vi "Sweep_Process.vi"(8 "错误输入（无错误）":errorcluster, 9 "MPM":refnum<k24>[](array[refnum]), 10 "TSL":refnum<k24>, 11 "SPU":refnum<k24>) -> (0 "error out":errorcluster, 1 "MPM out":refnum<k24>[](array[refnum]), 2 "TSL out":refnum<k24>, 3 "SPU out":refnum<k24>)   [LabVIEW 2017]
doc: "Sweep"
uses:
  D:/test/ILSTS/LV_IL/LV_IL_Sample_x64/DLL/InstrumentDLL.dll
  DLL/InstrumentDLL.dll
  Share/PowerMonitorType.vi
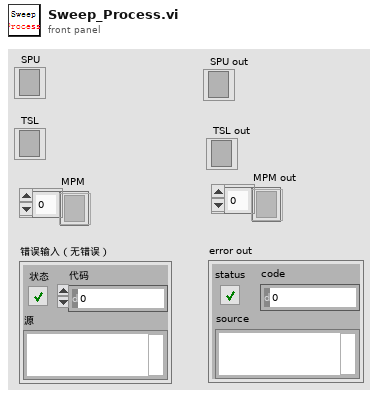
[diagram p1: front panel]
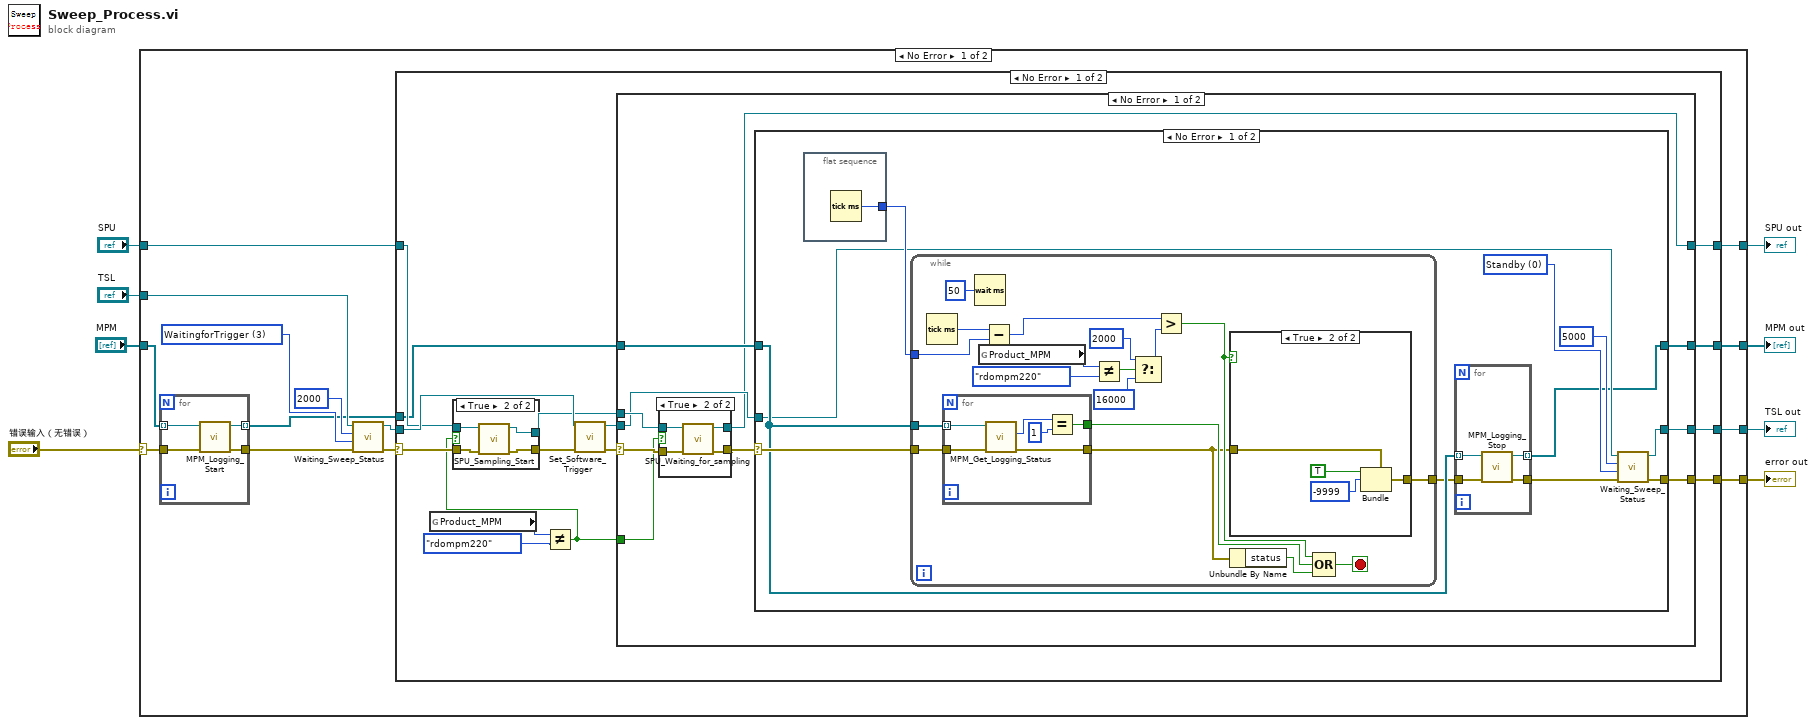
[diagram p0: block diagram]
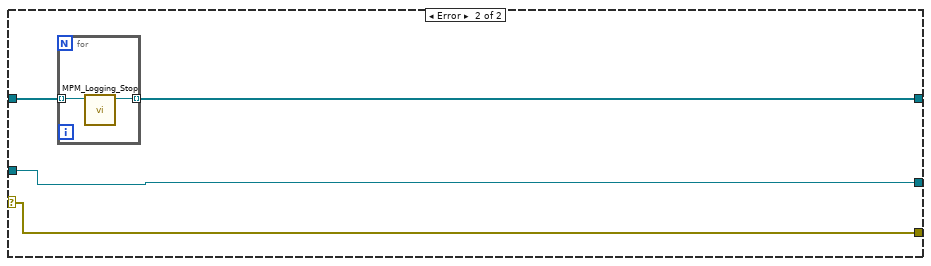
[diagram p5: hidden frame]
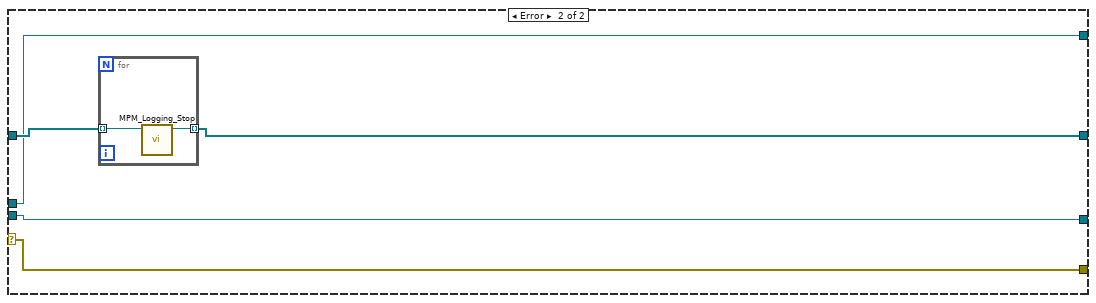
[diagram p6: hidden frame]
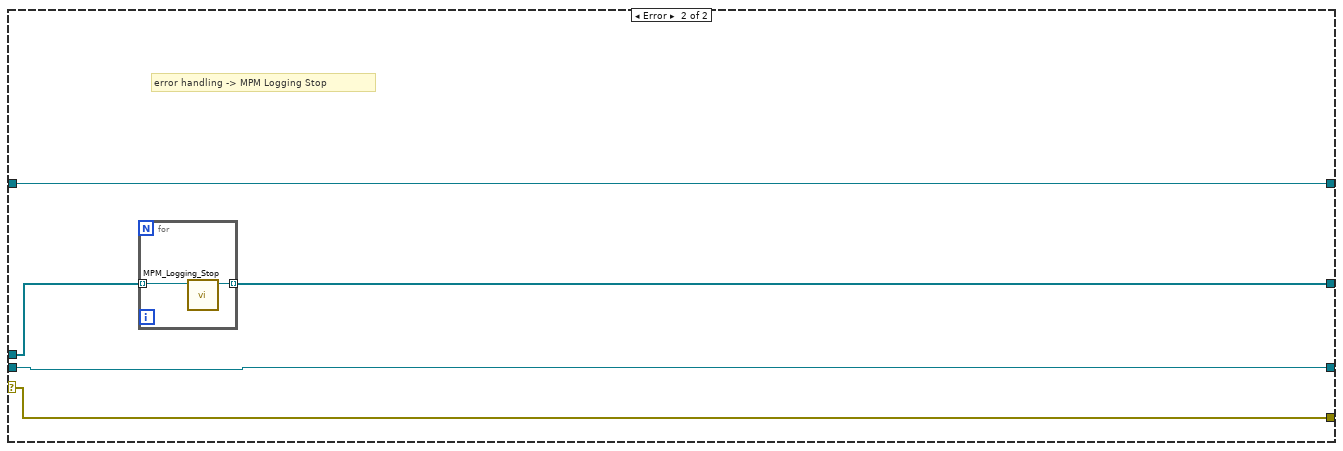
[diagram p7: hidden frame]
diagram:
  n1 = case shown="No Error" "错误输入（无错误）" {
    selector: "错误输入（无错误）" -> [w13 w132]
    tunnel: "SPU" -> [w22 w131]
    tunnel: "TSL" -> [w16 w130]
    tunnel: [w15 w132] -> w6
    tunnel: "MPM" -> [w14 w129]
    tunnel: [w12 w131] -> w3
    tunnel: [w11 w130] -> w2
    tunnel: [w9 w129] -> w1
    frame No Error {
      w19 = 3 items=["Standby", "Running", "Pausing", "WaitingforTrigger", "Returning"] ("status")
      n2 = for {
        tunnel: w14 -> [w128] mode=indexing
        tunnel: w13 -> [w127]
        tunnel: [w126] -> w17
        tunnel: [w125] -> w10 mode=indexing
        n3 = call "MPM_Logging_Start.vi"("error in (no error)"=w127, ".NET Reference in"=w128) -> ("error out"=w126:errorcluster, "Reference out"=w125:refnum<k24>)  [unwired: 8 in]
      }
      n4 = call "Waiting_Sweep_Status.vi"("error in (no error)"=w17, "status"=w19, "Wait time(msec)"=2000, ".NET Reference in"=w16) -> ("error out"=w20:errorcluster, "Reference out"=w21:refnum<k24>)  [unwired: 6 in]
      n5 = case shown="No Error" w20 {
        selector: w20 -> [w35 w121]
        tunnel: w21 -> [w36 w118]
        tunnel: w22 -> [w34 w120]
        tunnel: w10 -> [w33 w122]
        tunnel: [w29 w121] -> w15
        tunnel: [w28 w120] -> w12
        tunnel: [w27 w118] -> w11
        tunnel: [w26 w119] -> w9
        frame No Error {
          n6 = global read "PowerMonitorType.vi" "Product_MPM"() -> (w25:enum32{"rdompm210", "rdompm220"})
          n7 = Not Equal?(x=w25, y=enum32{"rdompm210", "rdompm220"}."rdompm220") -> (x != y?=w23:bool)
          n8 = case shown="True" w23 {
            tunnel: [w38 w43] -> w37
            tunnel: w35 -> [w38 w42]
            tunnel: w34 -> [w39 w41]
            tunnel: [w39 w40] -> w31
            frame False {
            }
            frame True {
              n9 = call "SPU_Sampling_Start.vi"("错误输入（无错误）"=w42, "引用"=w41) -> ("error IO"=w43:errorcluster, "引用输出"=w40:refnum<k24>)  [unwired: 7 in]
            }
          }
          n10 = call "Set_Software_Trigger.vi"("error in (no error)"=w37, ".NET Reference in"=w36) -> ("error out"=w32:errorcluster, "Reference out"=w30:refnum<k24>)  [unwired: 8 in]
          n11 = case shown="No Error" w32 {
            selector: w32 -> [w53 w114]
            tunnel: w33 -> [w50 w115]
            tunnel: w31 -> [w52 w113]
            tunnel: w30 -> [w49 w111]
            tunnel: [w48 w114] -> w29
            tunnel: [w47 w113] -> w28
            tunnel: [w46 w111] -> w27
            tunnel: [w45 w112] -> w26
            tunnel: w23 -> [w44 _]
            frame No Error {
              n12 = case shown="True" w44 {
                tunnel: w53 -> [w54 w59]
                tunnel: w52 -> [w55 w58]
                tunnel: [w54 w57] -> w51
                tunnel: [w55 w56] -> w47
                frame False {
                }
                frame True {
                  n13 = call "SPU_Waiting_for_sampling.vi"("错误输入（无错误）"=w59, "引用"=w58) -> ("error IO"=w57:errorcluster, "引用输出"=w56:refnum<k24>)  [unwired: 7 in]
                }
              }
              n14 = case shown="No Error" w51 {
                selector: w51 -> [w70 w107]
                tunnel: w50 -> [w68 w108]
                tunnel: w49 -> [w64 w105]
                tunnel: [w63 w107] -> w48
                tunnel: [w61 w105] -> w46
                tunnel: [w60 w106] -> w45
                frame No Error {
                  w66 = 0 items=["Standby", "Running", "Pausing", "WaitingforTrigger", "Returning"] ("status")
                  n15 = flat-sequence {
                    tunnel: [w75] -> w69
                    frame #0 {
                      n16 = Tick Count (ms)() -> (millisecond timer value=w75:u32)
                    }
                  }
                  n17 = while {
                    tunnel: w68 -> [w93]
                    tunnel: w70 -> [w92]
                    tunnel: w69 -> [w89]
                    tunnel: [w82] -> w62
                    stop <- w86 stop-if-true
                    n18 = Tick Count (ms)() -> (millisecond timer value=w90:u32)
                    n19 = for {
                      tunnel: w93 -> [w104] mode=indexing
                      tunnel: w92 -> [w103]
                      tunnel: [w100] -> w87
                      tunnel: [w99] -> w83
                      n20 = call "MPM_Get_Logging_Status.vi"("error in (no error)"=w103, ".NET Reference in"=w104) -> ("error out"=w99:errorcluster, "status out"=w102:i32)  [unwired: 6 in, 2 out]
                      n21 = Equal?(x=w102, y=1) -> (x = y?=w100:bool)
                    }
                    n22 = Wait (ms)(milliseconds to wait=u32 50 ("等待时间（毫秒）")) -> ()  [unwired: 1 out]
                    n23 = global read "PowerMonitorType.vi" "Product_MPM"() -> (w77:enum32{"rdompm210", "rdompm220"})
                    n24 = Subtract(x=w90, y=w89) -> (x-y=w88:u32)
                    n25 = Not Equal?(x=w77, y=enum32{"rdompm210", "rdompm220"}."rdompm220") -> (x != y?=w78:bool)
                    n26 = Select(t=u32 2000 ("y"), s=w78, f=u32 16000) -> (s? t:f=w79:u32)
                    n27 = Greater?(x=w88, y=w79) -> (0:w84:bool)
                    n28 = case shown="True" w84 {
                      tunnel: w83 -> [w94 w98]
                      tunnel: [w94 w95] -> w82
                      frame False {
                      }
                      frame True {
                        n29 = Bundle(cluster=w98, "status"=TRUE, "code"=-9999) -> (w95:errorcluster)  [unwired: 1 in]
                      }
                    }
                    n30 = Unbundle By Name(w83) -> ("status"=w85:bool)
                    n31 = Compound Arithmetic op=OR ("复合运算")(w84, w87, w85) -> (w86:bool)
                  }
                  n32 = for {
                    tunnel: w68 -> [w74] mode=indexing
                    tunnel: [w73] -> w67
                    tunnel: w62 -> [w72]
                    tunnel: [w71] -> w60 mode=indexing
                    n33 = call "MPM_Logging_Stop.vi"("error in (no error)"=w72, ".NET Reference in"=w74) -> ("error out"=w73:errorcluster, "Reference out"=w71:refnum<k24>)  [unwired: 8 in]
                  }
                  n34 = call "Waiting_Sweep_Status.vi"("error in (no error)"=w67, "status"=w66, "Wait time(msec)"=5000, ".NET Reference in"=w64) -> ("error out"=w63:errorcluster, "Reference out"=w61:refnum<k24>)  [unwired: 6 in]
                }
                frame Error {
                  n35 = for {
                    tunnel: w108 -> [w110] mode=indexing
                    tunnel: [w109] -> w106 mode=indexing
                    n36 = call "MPM_Logging_Stop.vi"(".NET Reference in"=w110) -> ("Reference out"=w109:refnum<k24>)  [unwired: 9 in, 1 out]
                  }
                }
              }
            }
            frame Error {
              n37 = for {
                tunnel: w115 -> [w117] mode=indexing
                tunnel: [w116] -> w112 mode=indexing
                n38 = call "MPM_Logging_Stop.vi"(".NET Reference in"=w117) -> ("Reference out"=w116:refnum<k24>)  [unwired: 9 in, 1 out]
              }
            }
          }
        }
        frame Error {
          # "error handling -> MPM Logging Stop"
          n39 = for {
            tunnel: w122 -> [w124] mode=indexing
            tunnel: [w123] -> w119 mode=indexing
            n40 = call "MPM_Logging_Stop.vi"(".NET Reference in"=w124) -> ("Reference out"=w123:refnum<k24>)  [unwired: 9 in, 1 out]
          }
        }
      }
    }
    frame Error {
    }
  }
  "error out" <- w6
  "SPU out" <- w3
  "TSL out" <- w2
  "MPM out" <- w1
